vi "com port dialog.vi"() -> (4 "VISA resource name out":refnum<visa-resource-name>, 6 "port opened":bool, 8 "version":dbl, 10 "message":string, 15 "error out":errorcluster)   [LabVIEW 2017]
uses:
  typedefs/commandType.ctl
panel:
  in  "open teensy":bool
  in  "VISA resource name":refnum<visa-resource-name>
  in  "select serial port automatically?":bool=TRUE
  in  "error in (no error)":errorcluster
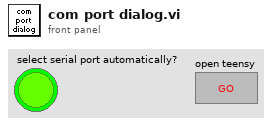
[diagram p1: front panel]
types:
  T1 = typedef "commandType.ctl" = enum16{"G - set gain", "C - activate coil", "D - deactivate coil", "L - set LED", "A - set AUTO", "V - set verbose", "T - set transmission", "R - get version", "Z - zero accelerometer"}
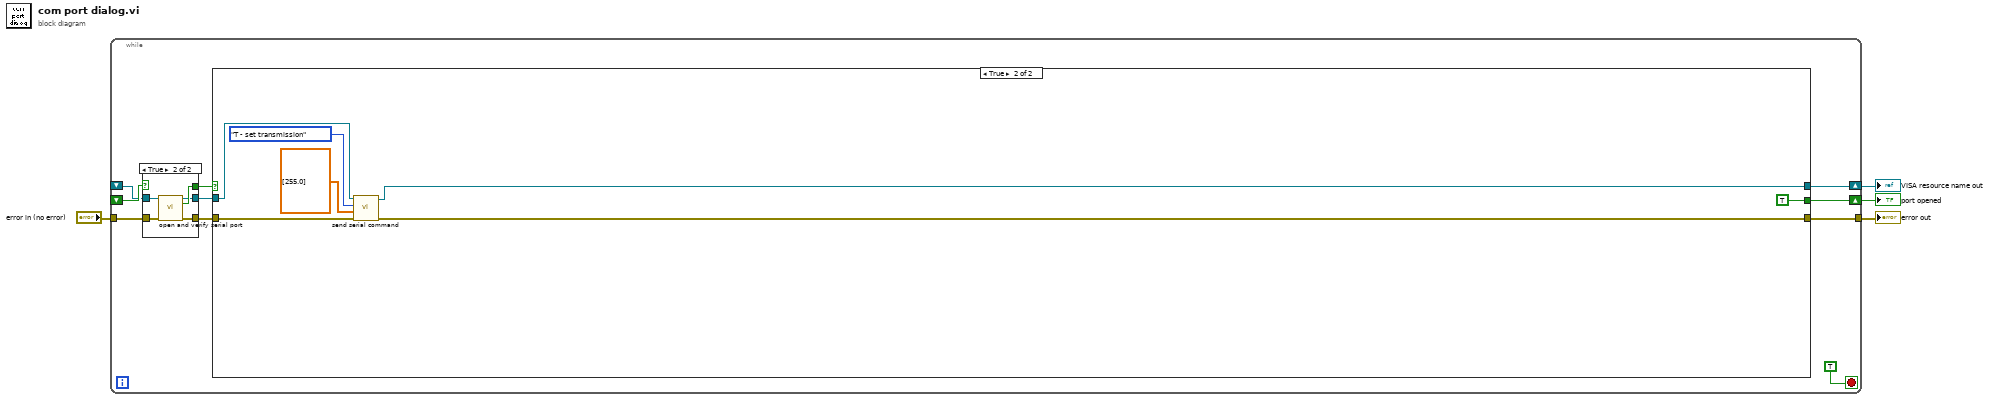
[diagram p0: block diagram]
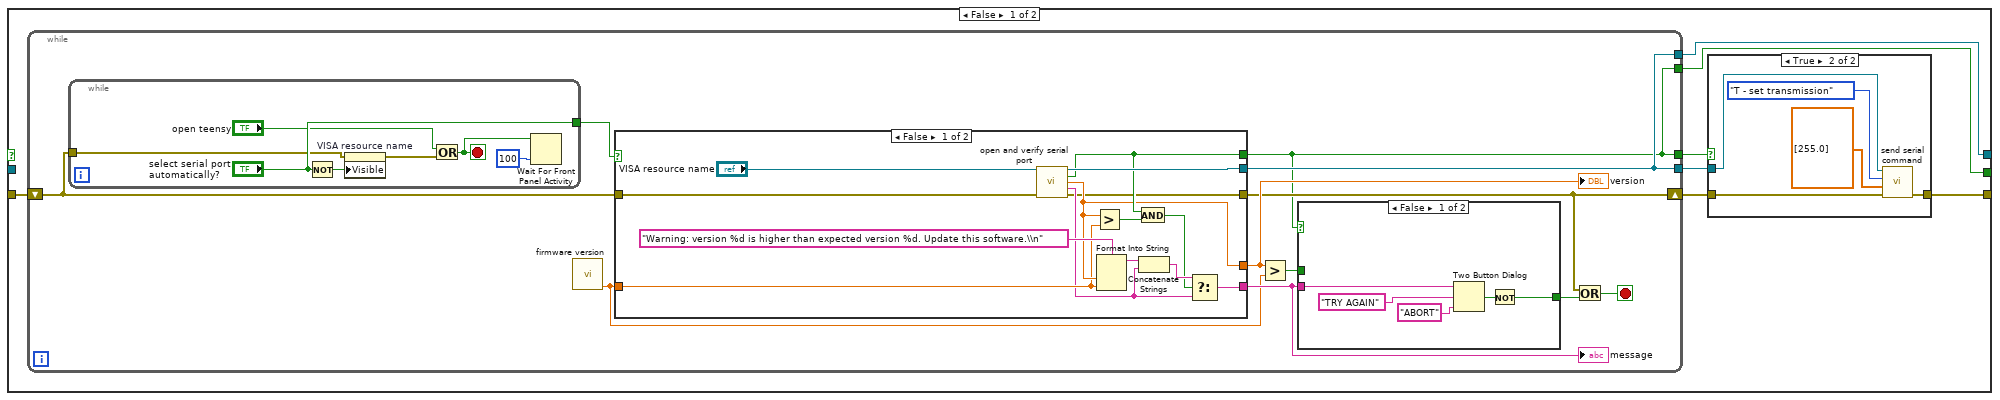
[diagram p2: hidden frame]
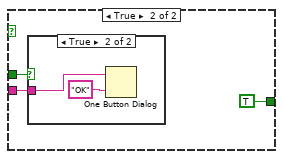
[diagram p4: hidden frame]
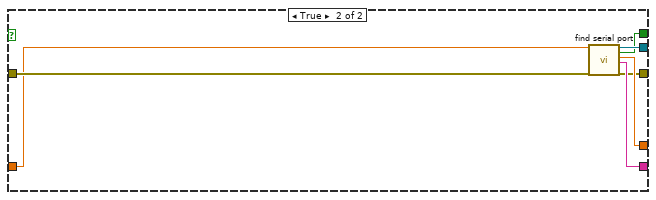
[diagram p6: hidden frame]
diagram:
  n1 = while {
    shift-right: [w13] -> w4
    shift-left: _ -> [w10]
    shift-right: [w12] -> w3
    shift-left: _ -> [w11]
    tunnel: "error in (no error)" -> [w9]
    tunnel: [w7] -> w1
    stop <- TRUE stop-if-true
    n2 = case shown="True" w11 {
      tunnel: w10 -> [_ w89]
      tunnel: w9 -> [w84 w88]
      tunnel: [w84 w87] -> w8
      tunnel: [_ w86] -> w6
      tunnel: [_ w85] -> w5
      frame False {
      }
      frame True {
        n3 = call "open and verify serial port.vi"("VISA resource name"=w89, "error in (no error)"=w88) -> ("VISA resource name out"=w85:refnum<visa-resource-name>, "port opened"=w86:bool, "error out"=w87:errorcluster)  [unwired: 9 in, 2 out]
      }
    }
    n4 = case shown="True" w6 {
      tunnel: [w18 w77] -> w13
      tunnel: [w17 TRUE ("port opened")] -> w12
      tunnel: w8 -> [w16 w79]
      tunnel: [w15 w78] -> w7
      tunnel: w5 -> [_ w80]
      frame False {
        n5 = while {
          shift-right: [w32] -> w21
          shift-left: w16 -> [w34]
          tunnel: [w29] -> w19
          tunnel: [w28] -> w20
          tunnel: [w29] -> w18
          tunnel: [w28] -> w17
          stop <- w33 stop-if-true
          n6 = while {
            tunnel: ["select serial port automatically?"] -> w38
            tunnel: w34 -> [w49]
            stop <- w51 stop-if-true
            n7 = Not(x="select serial port automatically?") -> (.not. x?=w55:bool)
            n8 = property on="VISA resource name" class="VISAName"(error in=w49, "Visible"=w55) -> (error out=w52:errorcluster)  [unwired: 1 in, 1 out]
            n9 = Or(x="open teensy", y=w52) -> (x .or. y?=w51:bool)
            n10 = Wait For Front Panel Activity(1:100 ("timeout ms (-1 never timeout)"), 3:w51) -> ()  [unwired: 1 in, 1 out]
          }
          n11 = call "firmware version.vi"() -> ("target firmware version"=w30:dbl)  [unwired: 11 in]
          n12 = case shown="False" w38 {
            tunnel: w34 -> [w69 w76]
            tunnel: [w67 w75] -> w29
            tunnel: [w63 w74] -> w28
            tunnel: [w62 w73] -> w37
            tunnel: [w57 w72] -> w35
            tunnel: w30 -> [w61 w71]
            tunnel: [w56 w70] -> w32
            frame False {
              n13 = call "open and verify serial port.vi"("VISA resource name"="VISA resource name", "error in (no error)"=w69) -> ("VISA resource name out"=w67:refnum<visa-resource-name>, "port opened"=w63:bool, "version"=w62:dbl, "message"=w59:string, "error out"=w56:errorcluster)  [unwired: 9 in]
              n14 = Greater?(x=w62, y=w61) -> (0:w64:bool)
              n15 = Format Into String(format string="Warning: version %d is higher than expected version %d. Update this software.\\n", w62, w61) -> (resulting string=w65:string)  [unwired: 2 in, 1 out]
              n16 = And(x=w63, y=w64) -> (x .and. y?=w58:bool)
              n17 = Concatenate Strings(w65, w59) -> (w60:string)
              n18 = Select(t=w60, s=w58, f=w59) -> (s? t:f=w57:string)
            }
            frame True {
              n19 = call "find serial port.vi"("target version"=w71, "error in (no error)"=w76) -> ("VISA resource name out"=w75:refnum<visa-resource-name>, "port opened"=w74:bool, "version"=w73:dbl, "message"=w72:string, "error out"=w70:errorcluster)  [unwired: 12 in, 1 out]
            }
          }
          "version" <- w37
          "message" <- w35
          n20 = Greater?(x=w37, y=w30) -> (0:w36:bool)
          n21 = case shown="False" w28 {
            tunnel: w36 -> [_ w46]
            tunnel: w35 -> [w43 w45]
            tunnel: [w39 TRUE ("T button?")] -> w31
            frame False {
              n22 = Two Button Dialog(message=w43, 1:"ABORT" ("button name (\"OK\")"), 2:"TRY AGAIN" ("T button name (\"OK\")")) -> (T button?=w40:bool)
              n23 = Not(x=w40) -> (.not. x?=w39:bool)
            }
            frame True {
              n24 = case shown="True" w46 {
                tunnel: w45 -> [_ w48]
                frame False {
                }
                frame True {
                  n25 = One Button Dialog(message=w48, button name ("OK")="OK") -> ()  [unwired: 1 out]
                }
              }
            }
          }
          n26 = Or(x=w32, y=w31) -> (x .or. y?=w33:bool)
        }
        n27 = case shown="True" w20 {
          tunnel: w21 -> [w22 w27]
          tunnel: w19 -> [_ w26]
          tunnel: [w22 w23] -> w15
          frame False {
          }
          frame True {
            n28 = call "send serial command.vi"("error in (no error)"=w27, "data"=dbl[] [255.0], "Command"=commandType."T - set transmission", "visa resource"=w26) -> ("error out"=w23:errorcluster)  [unwired: 5 in, 2 out]
          }
        }
      }
      frame True {
        n29 = call "send serial command.vi"("error in (no error)"=w79, "data"=dbl[] [255.0], "Command"=commandType."T - set transmission", "visa resource"=w80) -> ("error out"=w78:errorcluster, "VISA resource name out"=w77:refnum<visa-resource-name>)  [unwired: 5 in, 1 out]
      }
    }
  }
  "VISA resource name out" <- w4
  "port opened" <- w3
  "error out" <- w1
